vi "Py - density.vi"(7 "python in":refnum<k35>, 8 "error in":errorcluster, 11 "Z":i32) -> (0 "error out":errorcluster, 3 "density (g/cm3)":dbl, 5 "python out":refnum<k35>)   [LabVIEW 2023]
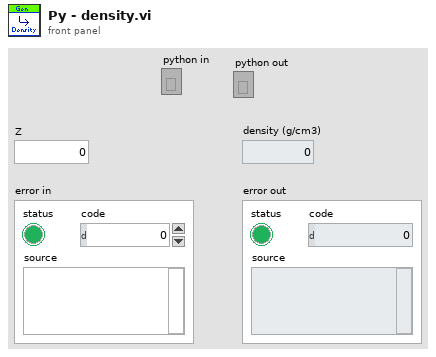
[diagram p1: front panel]
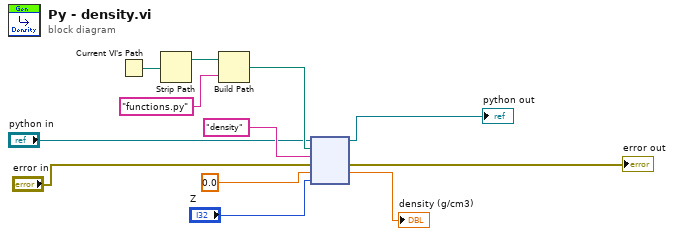
[diagram p0: block diagram]
diagram:
  n1 = Current VI's Path() -> (path=w11:path)
  n2 = Strip Path(path=w11) -> (stripped path=w10:path)  [unwired: 1 out]
  n3 = Build Path(base path=w10, name or relative path="functions.py") -> (appended path=w6:path)
  n4 = node("python in", w6, "density", "error in", 0.0, "Z") -> (→"python out":refnum<k35>, →"error out":errorcluster, →"density (g/cm3)":dbl)  [unwired: 1 in, 2 out]
